vi "Climb_Globals.vi"() -> ()   [LabVIEW 2019]
uses:
  Subsystems/Climb/Climb_Cluster.ctl
panel:
  in  "Climb_Execute_Notifier":refnum<notifier>
  in  "Climb_Set_Notifier":refnum<notifier>
  in  "Climb_Execute_Ref":string="Climb_Execute_Ref"
  in  "Climb_Set_Ref":string="Climb_Set_Ref"
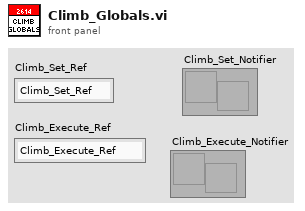
[diagram p1: front panel]
diagram:
